vi "GetParam.vi"(8 "error in (no error)":errorcluster caption="entrée d'erreur (pas d'erreur)", 11 "Multilabel_Confusion_Matrix.lvclass":refnum<class "Multilabel_Confusion_Matrix.lvclass">) -> (0 "error out":errorcluster caption="sortie d'erreur", 2 "multilabel_confusion_matrix":T1={"sample_weight"=[], "labels"={"dtype_labels"="None", "labels"=["None"]}, "samplewise"=FALSE}, 3 "Multilabel_Confusion_Matrix.lvclass":refnum<class "Multilabel_Confusion_Matrix.lvclass">)   [LabVIEW 2020, in "Multilabel_Confusion_Matrix.lvclass"]
doc: "Get Parameters"
uses:
  Multilabel_Confusion_Matrix.lvclass
  Multilabel_Confusion_Matrix.lvclass/Multilabel_Confusion_Matrix.ctl
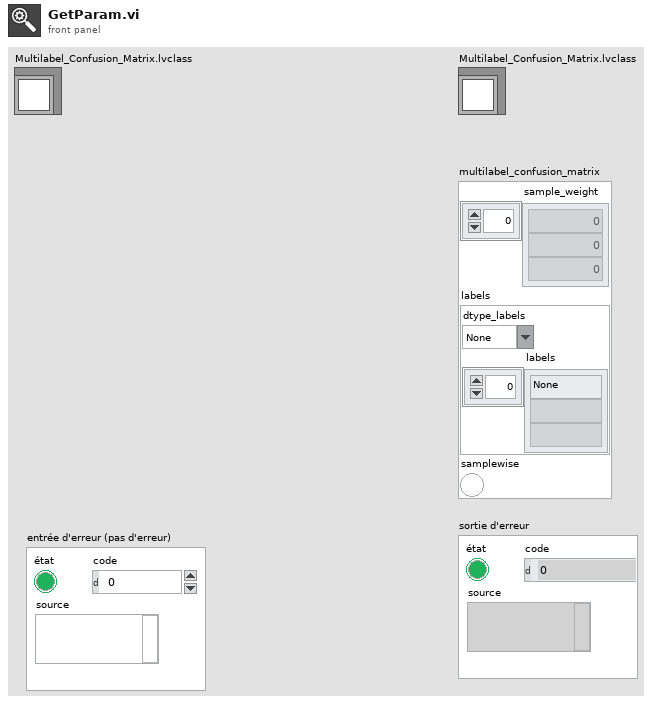
[diagram p1: front panel]
types:
  T1 = cluster{"sample_weight":dbl[], "labels":cluster{"dtype_labels":string, "labels":string[]}, "samplewise":bool}
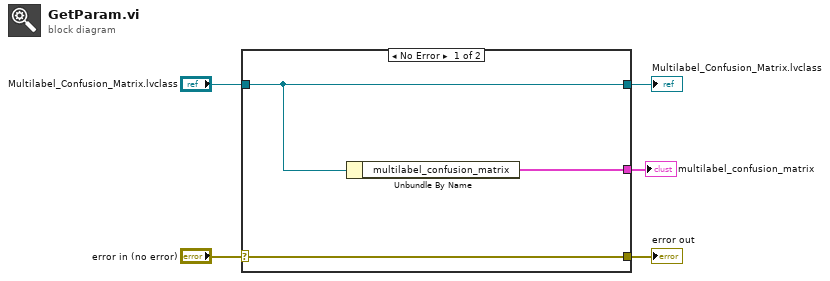
[diagram p0: block diagram]
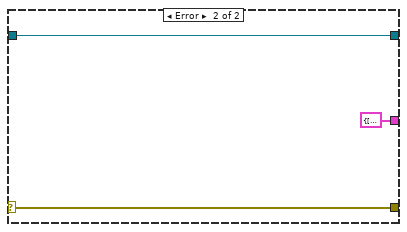
[diagram p2: hidden frame]
diagram:
  n1 = case shown="No Error" "error in (no error)" {
    selector: "error in (no error)" -> [w8 w10]
    tunnel: [w8 w10] -> w4
    tunnel: [w7 w11] -> w2
    tunnel: "Multilabel_Confusion_Matrix.lvclass" -> [w7 w11]
    tunnel: [w6 T1 {"sample_weight"=[], "labels"={"dtype_labels"="", "labels"=[]}, "samplewise"=FALSE} ("multilabel_confusion_matrix")] -> w1
    frame No Error {
      n2 = Unbundle By Name(w7) -> ("multilabel_confusion_matrix"=w6:T1)
    }
    frame Error {
    }
  }
  "error out" <- w4
  "Multilabel_Confusion_Matrix.lvclass" <- w2
  "multilabel_confusion_matrix" <- w1
